vi "Begin.vi"() -> (0 "error out":errorcluster)   [LabVIEW 2013]
doc: "Called before other user functions, this VI is expected to open initial I/O refnums, load in file data, and do all program initialization. Notice that the <B>error out</B> terminal is simply used for data flow. Wiring it to other structures or subVIs ensures that this VI runs first."
uses:
  <vilib>/Rock Robotics/WPI/SafetyOutput/WPI_SafetyOutputConfigMenu.ctl
  <vilib>/Rock Robotics/WPI/DriverStation/WPI_DriverStationRobotMode2.ctl
  <vilib>/Rock Robotics/WPI/Joystick/WPI_JoystickDeviceEnum.ctl
  <vilib>/Rock Robotics/SystemInterfaces/DIO/FPGA_DIOPWMChannel.ctl
  <vilib>/Rock Robotics/SystemInterfaces/AI/FPGA_AIGyroChannel.ctl
  Program Files (x86)/National Instruments/LabVIEW 2013/examples/FRC/I2C/ADXL345 I2C/Driver/ADXL345 I2C Range.ctl
  <vilib>/Rock Robotics/SystemInterfaces/Typedef/FPGA_TypedefDigitalModule.ctl
  <vilib>/Rock Robotics/SystemInterfaces/DIO/FPGA_DIOChannel.ctl
  <vilib>/Rock Robotics/SystemInterfaces/DIO/FPGA_DIORelayChannel.ctl
  <vilib>/Rock Robotics/WPI/Relay/WPI_RelayDirection.ctl
  Robot Global Data.vi
  <vilib>/Rock Robotics/WPI/RobotDrive/WPI_RobotDriveOpen2MotorWithJaguar.vi
  <vilib>/Rock Robotics/WPI/Counter/WPI_CounterDigitalInputToDigitalSource.vi
  <vilib>/Rock Robotics/WPI/MotorControl/WPI_MotorControlOpen Talon.vi
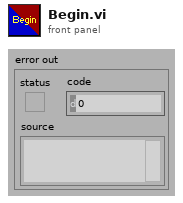
[diagram p1: front panel]
types:
  T1 = typedef "FPGA_DIOPWMChannel.ctl" = enum8{"PWM 1", "PWM 2", "PWM 3", "PWM 4", "PWM 5", "PWM 6", "PWM 7", "PWM 8", "PWM 9", "PWM 10", "Invalid"}
  T2 = typedef "FPGA_DIORelayChannel.ctl" = enum8{"Relay 1", "Relay 2", "Relay 3", "Relay 4", "Relay 5", "Relay 6", "Relay 7", "Relay 8", "Invalid"}
  T3 = typedef "WPI_RelayDirection.ctl" = enum16{"Both directions", "Forward only", "Reverse only"}
  T4 = typedef "FPGA_DIOChannel.ctl" = enum8{"DIO 1", "DIO 2", "DIO 3", "DIO 4", "DIO 5", "DIO 6", "DIO 7", "DIO 8", "DIO 9", "DIO 10", "DIO 11", "DIO 12", "DIO 13", "DIO 14", "Invalid"}
  T5 = typedef "FPGA_TypedefDigitalModule.ctl" = enum16{"Digital Module 1", "Digital Module 2"}
  T6 = typedef "ADXL345 I2C Range.ctl" = u8
  T7 = typedef "FPGA_AIGyroChannel.ctl" = enum8{"AI 1", "AI 2", "Invalid"}
  T8 = typedef "WPI_JoystickDeviceEnum.ctl" = enum16{"USB 1", "USB 2", "USB 3", "USB 4", "Kinect 1", "Kinect 2"}
  T9 = typedef "WPI_DriverStationRobotMode2.ctl" = enum16{"Autonomous Disabled", "Autonomous Enabled", "Teleop Disabled", "Teleop Enabled", "Timeout", "Finish", "Test Disabled", "Test Enabled"}
  T10 = typedef "WPI_SafetyOutputConfigMenu.ctl" = enum16{"Enable", "Disable"}
  T11 = typedef "WPI_JoystickDevRef.ctl" = cluster{"Device":T8}
  T12 = typedef "WPI_RobotDriveDevRef.ctl" = cluster{"DevStatus":errorcluster, "Motors[]":T13[], "Square Inputs":bool, "Max Output":dbl, "Isochronous":bool}
  T13 = typedef "WPI_MotorControlDeviceRef.ctl" = cluster{"DeviceStatus":errorcluster, "Type":enum16{"PWM", "CAN"}, "PWM":cluster{"Digital Module":T5, "PWM Channel":T1, "DeadBand":T14}, "CAN":cluster{"Device Number":u8, "Control Mode":T15, "Semaphore":T16, "Max Vout":dbl}, "Invert":bool, "TransformRef":T17, "InvTransformRef":T17}
  T14 = typedef "WPI_PWMDeadband.ctl" = cluster{"Name":string, "maxPositivePwm":i32, "minPositivePwm":i32, "centerPwm":i32, "maxNegativePwm":i32, "minNegativePwm":i32, "angularRange":u16}
  T15 = typedef "WPI_CANJaguar_ControlMode.ctl" = enum8{"Percent VBus", "Current", "Speed", "Position", "Voltage"}
  T16 = typedef "Semaphore RefNum" = refnum<k1>
  T17 = typedef "WPI_PWMTransform_ConPane.ctl" = refnum<vi>
  T18 = typedef "WPI_ServoDeviceRef.ctl" = cluster{"DeviceStatus":errorcluster, "Digital Module":T5, "PWM Channel":T1, "DeadBand":T14}
  T19 = typedef "WPI_I2CDevRef.ctl" = cluster{"DevStatus":errorcluster, "Digital Module":T5, "Device Address":u8}
  T20 = typedef "WPI_RelayDevRef.ctl" = cluster{"DevStatus":errorcluster, "Relay Channel":T2, "Digital Module":T5, "Relay Direction":T3}
  T21 = typedef "WPI_GyroDevRef.ctl" = cluster{"DevStatus":errorcluster, "Analog Module":T22, "Analog Channel":T23, "Offset":dbl, "Gain (VoltsPerDegree/Second)":dbl}
  T22 = typedef "FPGA_TypedefAnalogModule.ctl" = enum16{"Analog Module 1", "Analog Module 2"}
  T23 = typedef "FPGA_AIChannel.ctl" = enum8{"AI 1", "AI 2", "AI 3", "AI 4", "AI 5", "AI 6", "AI 7", "AI 8", "Invalid"}
  T24 = typedef "WPI_DigitalInputDevRef.ctl" = cluster{"DevStatus":errorcluster, "DIO Channel":T4, "Digital Module":T5}
  T25 = typedef "FPGA_CounterEncoderSourceConvertionLVSourceType.ctl" = cluster{"DevStatus":errorcluster, "AnalogTriggerMode?":bool, "DigitalMode":cluster{"Digital Module":T5, "DIO Channel":T26}, "AnalogTriggerMode":cluster{"AnalogTriggerIndex":T27, "OutputType":T28}}
  T26 = typedef "FPGA_DIODigitalSourceChannel.ctl" = enum8{"DIO 1", "DIO 2", "DIO 3", "DIO 4", "DIO 5", "DIO 6", "DIO 7", "DIO 8", "DIO 9", "DIO 10", "DIO 11", "DIO 12", "DIO 13", "DIO 14", "Disabled"}
  T27 = typedef "FPGA_AnalogTriggerIndex.ctl" = enum8{"Trig 0", "Trig 1", "Trig 2", "Trig 3", "Trig 4", "Trig 5", "Trig 6", "Trig 7", "Invalid"}
  T28 = typedef "FPGA_AnalogTriggerOutType.ctl" = enum16{"InWindow", "TriggerState", "Rising", "Falling"}
  T29 = typedef "WPI_EncoderDevRef.ctl" = cluster{"DevStatus":errorcluster, "EncoderIndex":T30, "CounterIndex":T31, "DistancePerCount":dbl, "Decoding Type":T32}
  T30 = typedef "FPGA_EncoderIdx.ctl" = enum8{"Enc 0", "Enc 1", "Enc 2", "Enc 3", "Invalid"}
  T31 = typedef "FPGA_CounterCtrSystemIndex.ctl" = enum8{"Ctr 0", "Ctr 1", "Ctr 2", "Ctr 3", "Ctr 4", "Ctr 5", "Ctr 6", "Ctr 7", "Invalid"}
  T32 = typedef "WPI_EncoderType.ctl" = enum16{"1x", "2x", "4x"}
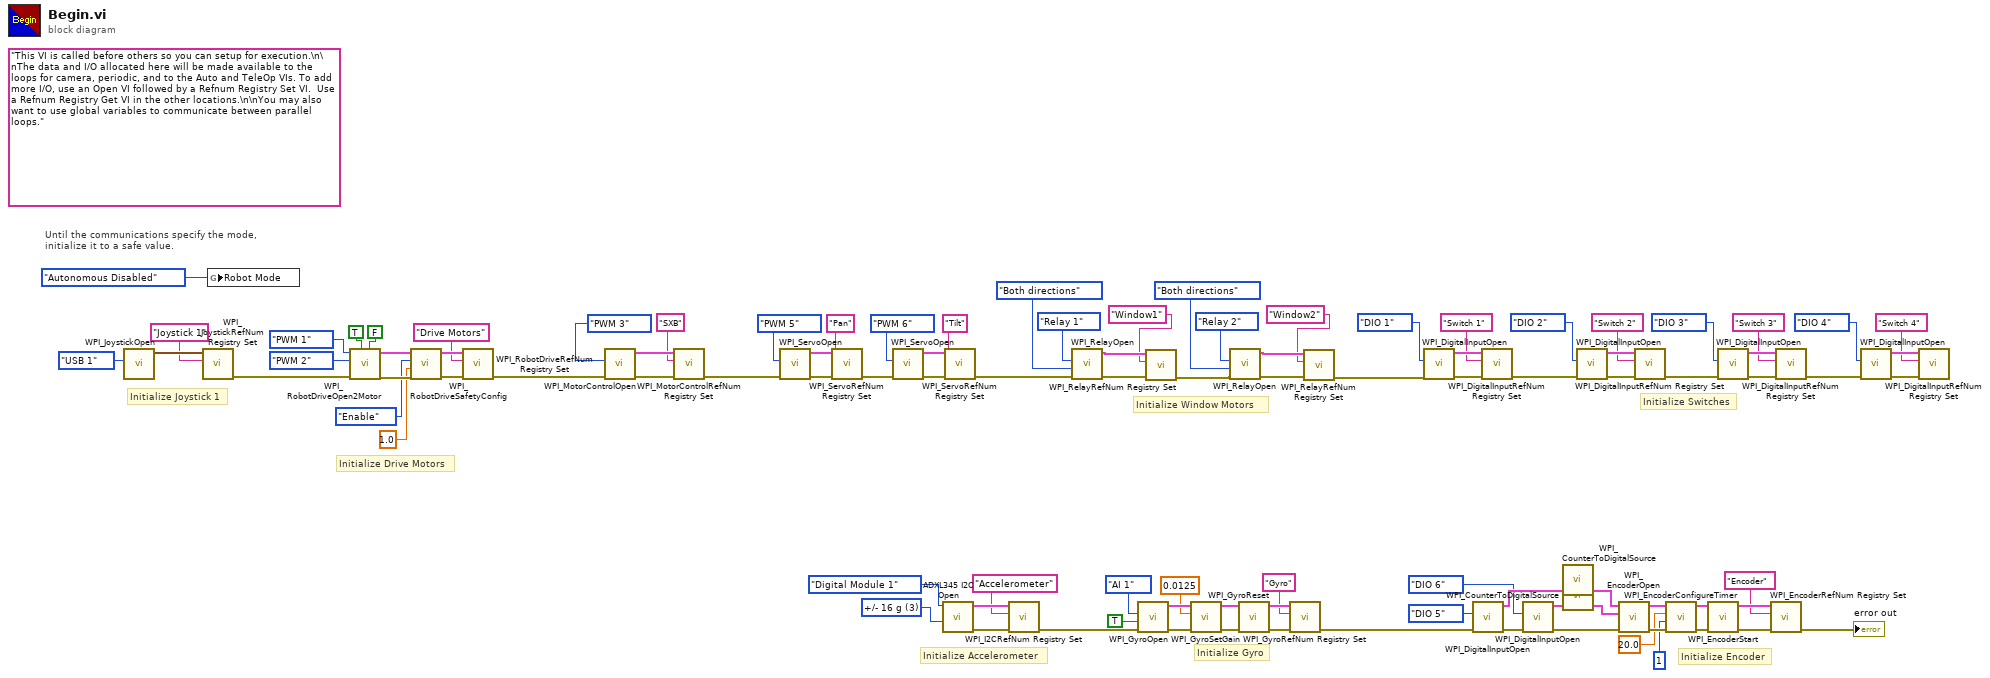
[diagram p0: block diagram]
diagram:
  w80 = T6 3 items=["+/- 2 g", "+/- 4 g", "+/- 8 g", "+/- 16 g"] ("Range")
  (unwired) "This VI is called before others so you can setup for execution.\n\nThe data and I/O allocated here will be made available to the loops for camera, periodic, and to the Auto and TeleOp VIs. To add more I/O, use an Open VI followed by a Refnum Registry Set VI.  Use a Refnum Registry Get VI in the other locations.\n\nYou may also want to use global variables to communicate between parallel loops."
  # "Initialize Window Motors"
  # "Initialize Switches"
  # "Initialize Encoder"
  # "Initialize Gyro"
  # "Initialize Accelerometer"
  # "Initialize Joystick 1"
  # "Until the communications specify the mode,\ninitialize it to a safe value."
  # "Initialize Drive Motors"
  n1 = call <vilib>:"WPI_JoystickOpen.vi"("JoystickDevice"=WPI_JoystickDeviceEnum."USB 1") -> ("JoystickDevRef"=w97:T11)  [unwired: 10 in]
  n2 = call <vilib>:"WPI_JoystickRefNum Registry Set.vi"("refnum name"="Joystick 1", "JoystickDevRef"=w97) -> ("error out"=w90:errorcluster)  [unwired: 8 in, 1 out]
  n3 = global write "Robot Global Data.vi" "Robot Mode"(WPI_DriverStationRobotMode2."Autonomous Disabled" ("Robot Mode")) -> ()
  n4 = call-poly <vilib>:"WPI_RobotDriveOpen2Motor.vi"("Right Motor Inverted"=FALSE, "Left Motor Inverted"=TRUE, "error in (no error)"=w90, "Right Motor"=FPGA_DIOPWMChannel."PWM 2", "Left Motor"=FPGA_DIOPWMChannel."PWM 1") -> ("error out"=w91:errorcluster, "RobotDriveDevRef"=w92:T12)  [unwired: 5 in]
  n5 = call <vilib>:"WPI_RobotDriveSafetyConfig.vi"("error in (no error)"=w91, "timeout (s)"=1.0, "mode"=WPI_SafetyOutputConfigMenu."Enable", "RobotDriveDevRef"=w92) -> ("error out"=w94:errorcluster, "RobotDriveDevRef"=w95:T12)  [unwired: 6 in]
  n6 = call <vilib>:"WPI_RobotDriveRefNum Registry Set.vi"("error in (no error)"=w94, "refnum name"="Drive Motors", "RobotDriveDevRef"=w95) -> ("error out"=w46:errorcluster)  [unwired: 8 out]
  n7 = call-poly <vilib>:"WPI_MotorControlOpen.vi"("error in (no error)"=w46, "PWM Channel"=FPGA_DIOPWMChannel."PWM 3") -> ("error out"=w44:errorcluster, "MotorControlDeviceRef"=w45:T13)  [unwired: 8 in]
  n8 = call <vilib>:"WPI_MotorControlRefNum Registry Set.vi"("error in (no error)"=w44, "refnum name"="SXB", "MotorControlDevRef"=w45) -> ("error out"=w2:errorcluster)  [unwired: 7 in, 1 out]
  n9 = call <vilib>:"WPI_ServoOpen.vi"("error in (no error)"=w2, "PWM Channel"=FPGA_DIOPWMChannel."PWM 5") -> ("error out"=w10:errorcluster, "ServoDeviceRef"=w9:T18)  [unwired: 8 in]
  n10 = call <vilib>:"WPI_ServoRefNum Registry Set.vi"("error in (no error)"=w10, "refnum name"="Pan", "ServoDeviceRef"=w9) -> ("error out"=w3:errorcluster)  [unwired: 7 in, 1 out]
  n11 = call <vilib>:"WPI_ServoOpen.vi"("error in (no error)"=w3, "PWM Channel"=FPGA_DIOPWMChannel."PWM 6") -> ("error out"=w6:errorcluster, "ServoDeviceRef"=w5:T18)  [unwired: 8 in]
  n12 = call "ADXL345 I2C Open.vi"("Range"=w80, "DIO Module (Module 1)"=FPGA_TypedefDigitalModule."Digital Module 1") -> ("error out"=w78:errorcluster, "I2CDevRef"=w77:T19)  [unwired: 2 in, 6 out]
  n13 = call <vilib>:"WPI_ServoRefNum Registry Set.vi"("error in (no error)"=w6, "refnum name"="Tilt", "ServoDeviceRef"=w5) -> ("error out"=w1:errorcluster)  [unwired: 7 in, 1 out]
  n14 = call <vilib>:"WPI_I2CRefNum Registry Set.vi"("error in (no error)"=w78, "refnum name"="Accelerometer", "I2CDevRef"=w77) -> ("error out"=w75:errorcluster)  [unwired: 7 in, 1 out]
  n15 = call <vilib>:"WPI_RelayOpen.vi"("error in (no error)"=w1, "Relay Direction"=WPI_RelayDirection."Both directions", "Relay Channel"=FPGA_DIORelayChannel."Relay 1") -> ("error out"=w19:errorcluster, "RelayDevRef"=w21:T20)  [unwired: 7 in]
  n16 = call <vilib>:"WPI_GyroOpen.vi"("error in (no error)"=w75, "Calibrate On Open"=TRUE, "Analog Channel"=FPGA_AIGyroChannel."AI 1") -> ("error out"=w74:errorcluster, "GyroDevRef"=w82:T21)  [unwired: 6 in, 1 out]
  n17 = call <vilib>:"WPI_RelayRefNum Registry Set.vi"("error in (no error)"=w19, "refnum name"="Window1", "RelayDevRef"=w21) -> ("error out"=w13:errorcluster)  [unwired: 7 in, 1 out]
  n18 = call <vilib>:"WPI_GyroSetGain.vi"("error in (no error)"=w74, "Gain (VoltsPerDegree/Second)"=0.0125, "GyroDevRef"=w82) -> ("error out"=w73:errorcluster, "GyroDevRef"=w79:T21)  [unwired: 7 out]
  n19 = call <vilib>:"WPI_RelayOpen.vi"("error in (no error)"=w13, "Relay Direction"=WPI_RelayDirection."Both directions", "Relay Channel"=FPGA_DIORelayChannel."Relay 2") -> ("error out"=w14:errorcluster, "RelayDevRef"=w16:T20)  [unwired: 7 in]
  n20 = call <vilib>:"WPI_GyroReset.vi"("error in (no error)"=w73, "GyroDevRef"=w79) -> ("error out"=w71:errorcluster, "GyroDevRef"=w72:T21)  [unwired: 8 in]
  n21 = call <vilib>:"WPI_GyroRefNum Registry Set.vi"("error in (no error)"=w71, "refnum name"="Gyro", "GyroDevRef"=w72) -> ("error out"=w66:errorcluster)  [unwired: 7 in, 1 out]
  n22 = call <vilib>:"WPI_RelayRefNum Registry Set.vi"("error in (no error)"=w14, "refnum name"="Window2", "RelayDevRef"=w16) -> ("error out"=w12:errorcluster)  [unwired: 7 in, 1 out]
  n23 = call <vilib>:"WPI_DigitalInputOpen.vi"("error in (no error)"=w12, "DIO Channel"=FPGA_DIOChannel."DIO 1") -> ("error out"=w30:errorcluster, "DigitalInputDevRef"=w43:T24)  [unwired: 8 in]
  n24 = call <vilib>:"WPI_DigitalInputOpen.vi"("error in (no error)"=w66, "DIO Channel"=FPGA_DIOChannel."DIO 5") -> ("error out"=w59:errorcluster, "DigitalInputDevRef"=w62:T24)  [unwired: 8 in]
  n25 = call <vilib>:"WPI_DigitalInputRefNum Registry Set.vi"("error in (no error)"=w30, "refnum name"="Switch 1", "DigitalInputDevRef"=w43) -> ("error out"=w29:errorcluster)  [unwired: 7 in, 1 out]
  n26 = call <vilib>:"WPI_DigitalInputOpen.vi"("error in (no error)"=w59, "DIO Channel"=FPGA_DIOChannel."DIO 6") -> ("error out"=w58:errorcluster, "DigitalInputDevRef"=w63:T24)  [unwired: 8 in]
  n27 = call-poly <vilib>:"WPI_CounterToDigitalSource.vi"("DigitalInputDevRef"=w62) -> ("Digital Source"=w55:T25)  [unwired: 6 in]
  n28 = call-poly <vilib>:"WPI_CounterToDigitalSource.vi"("DigitalInputDevRef"=w63) -> ("Digital Source"=w64:T25)  [unwired: 6 in]
  n29 = call <vilib>:"WPI_DigitalInputOpen.vi"("error in (no error)"=w29, "DIO Channel"=FPGA_DIOChannel."DIO 2") -> ("error out"=w28:errorcluster, "DigitalInputDevRef"=w39:T24)  [unwired: 8 in]
  n30 = call <vilib>:"WPI_EncoderOpen.vi"("error in (no error)"=w58, "BSource"=w64, "ASource"=w55) -> ("error out"=w57:errorcluster, "EncoderDevRef"=w61:T29)  [unwired: 7 in]
  n31 = call <vilib>:"WPI_DigitalInputRefNum Registry Set.vi"("error in (no error)"=w28, "refnum name"="Switch 2", "DigitalInputDevRef"=w39) -> ("error out"=w27:errorcluster)  [unwired: 7 in, 1 out]
  n32 = call <vilib>:"WPI_EncoderConfigureTimer.vi"("error in (no error)"=w57, "Number Samples to Average"=u8 1, "Minimum Rate"=20.0, "EncoderDevRef"=w61) -> ("error out"=w56:errorcluster, "EncoderDevRef"=w60:T29)  [unwired: 6 out]
  n33 = call <vilib>:"WPI_EncoderStart.vi"("error in (no error)"=w56, "EncoderDevRef"=w60) -> ("error out"=w52:errorcluster, "EncoderDevRef"=w51:T29)  [unwired: 8 in]
  n34 = call <vilib>:"WPI_DigitalInputOpen.vi"("error in (no error)"=w27, "DIO Channel"=FPGA_DIOChannel."DIO 3") -> ("error out"=w26:errorcluster, "DigitalInputDevRef"=w36:T24)  [unwired: 8 in]
  n35 = call <vilib>:"WPI_EncoderRefNum Registry Set.vi"("error in (no error)"=w52, "refnum name"="Encoder", "EncoderDevRef"=w51) -> ("error out"=→"error out":errorcluster)  [unwired: 7 in, 1 out]
  n36 = call <vilib>:"WPI_DigitalInputRefNum Registry Set.vi"("error in (no error)"=w26, "refnum name"="Switch 3", "DigitalInputDevRef"=w36) -> ("error out"=w25:errorcluster)  [unwired: 7 in, 1 out]
  n37 = call <vilib>:"WPI_DigitalInputOpen.vi"("error in (no error)"=w25, "DIO Channel"=FPGA_DIOChannel."DIO 4") -> ("error out"=w24:errorcluster, "DigitalInputDevRef"=w33:T24)  [unwired: 8 in]
  n38 = call <vilib>:"WPI_DigitalInputRefNum Registry Set.vi"("error in (no error)"=w24, "refnum name"="Switch 4", "DigitalInputDevRef"=w33) -> ()  [unwired: 7 in, 2 out]
